vi "FT_Open_Device_By_Description.vi"(8 "error in (no error)":errorcluster, 11 "Device Description":string) -> (0 "error out":errorcluster, 1 "FT_Status":u32(ring) items=["FT_OK", "FT_INVALID_HANDLE", "FT_DEVICE_NOT_FOUND", "FT_DEVICE_NOT_OPENED", "FT_IO_ERROR", "FT_INSUFFICIENT_RESOURCES", "FT_INVALID_PARAMETER", "FT_INVALID_BAUD_RATE", "FT_DEVICE_NOT_OPENED_FOR_ERASE", "FT_DEVICE_NOT_OPENED_FOR_WRITE", "FT_FAILED_TO_WRITE_DEVICE", "FT_EEPROM_READ_FAILED", "FT_EEPROM_WRITE_FAILED", "FT_EEPROM_ERASE_FAILED", "FT_EEPROM_NOT_PRESENT", "FT_EEPROM_NOT_PROGRAMMED", "FT_INVALID_ARGS", "FT_NOT_SUPPORTED", "FT_OTHER_ERROR"], 3 "Handle":u64)   [LabVIEW 2018]
uses:
  FTD2XX.dll
panel:
  in  "device":i32
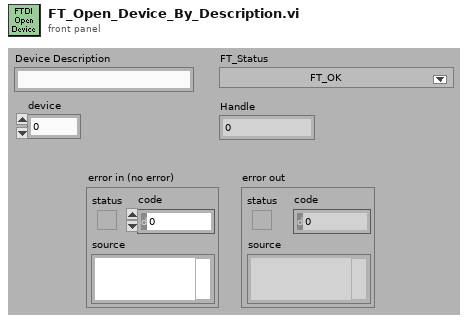
[diagram p1: front panel]
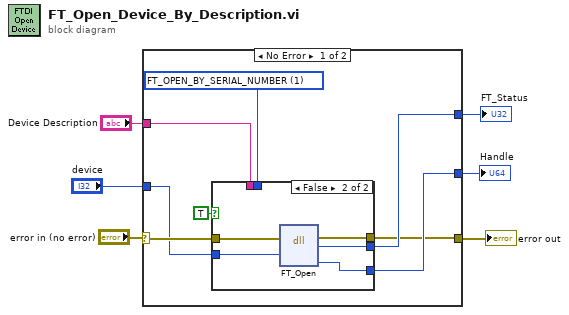
[diagram p0: block diagram]
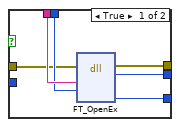
[diagram p2: hidden frame]
diagram:
  n1 = case shown="No Error" "error in (no error)" {
    selector: "error in (no error)" -> [w10 w26]
    tunnel: [w14 _] -> w6
    tunnel: [w13 _] -> w5
    tunnel: "Device Description" -> [w12 _]
    tunnel: [w9 w26] -> w2
    tunnel: "device" -> [w7 _]
    frame No Error {
      w11 = u32 1 items=["FT_OPEN_BY_SERIAL_NUMBER"=1, "FT_OPEN_BY_DESCRIPTION"=2, "FT_OPEN_BY_LOCATION"=4] ("Flags")
      n2 = case shown="False" TRUE {
        tunnel: [w20 w25] -> w14
        tunnel: [w19 w24] -> w13
        tunnel: w12 -> [w18 _]
        tunnel: w11 -> [w17 _]
        tunnel: w10 -> [w16 w23]
        tunnel: [w15 w22] -> w9
        tunnel: w7 -> [_ w21]
        frame True {
          n3 = dll-call lib="FTD2XX.dll" fn="FT_OpenEx"(error in=w16, "DeviceDescription"=w18, "Flags"=w17) -> (error out=w15:errorcluster, "FT_Status"=w19:u32, "Handle"=w20:u64)  [unwired: 5 in, 1 out]
        }
        frame False {
          n4 = dll-call lib="FTD2XX.dll" fn="FT_Open"(error in=w23, "device"=w21) -> (error out=w22:errorcluster, "FT_Status"=w24:u32, "Handle"=w25:u64)  [unwired: 4 in, 1 out]
        }
      }
    }
    frame Error {
    }
  }
  "Handle" <- w6
  "FT_Status" <- w5
  "error out" <- w2
